vi "Block Crafter.vi"(9 "In Items/t":ext) -> (3 "Out Items/t":ext)   [LabVIEW 2023]
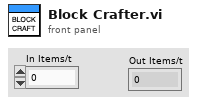
[diagram p1: front panel]
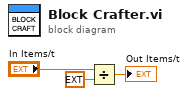
[diagram p0: block diagram]
diagram:
  n1 = Divide(x="In Items/t", y=ext 9.0) -> (x/y=→"Out Items/t":ext)
